vi "GFITS_GetHeaderArray.vi"(0 "file":path, 5 "mext":bool, 7 "number of Extensions":u16, 9 "readmode":string, 11 "error in (no error)":errorcluster, 12 "def_timing":string="after", 13 "headers":bool=TRUE) -> (4 "number of before":i32[](array[numeric]), 6 "After keys":string[][][](array[string]), 8 "number of after keywords":i32[](array[numeric]), 10 "totkeys":i32, 14 "before Keywords":string[][][](array[string]), 15 "error out":errorcluster)   [LabVIEW 2016]
uses:
  DBSHAND/private/vis/DatabaseHand_RefNum.ctl
  GFITS_Gbls.vi
panel:
  in  "Database RefNum in":T1
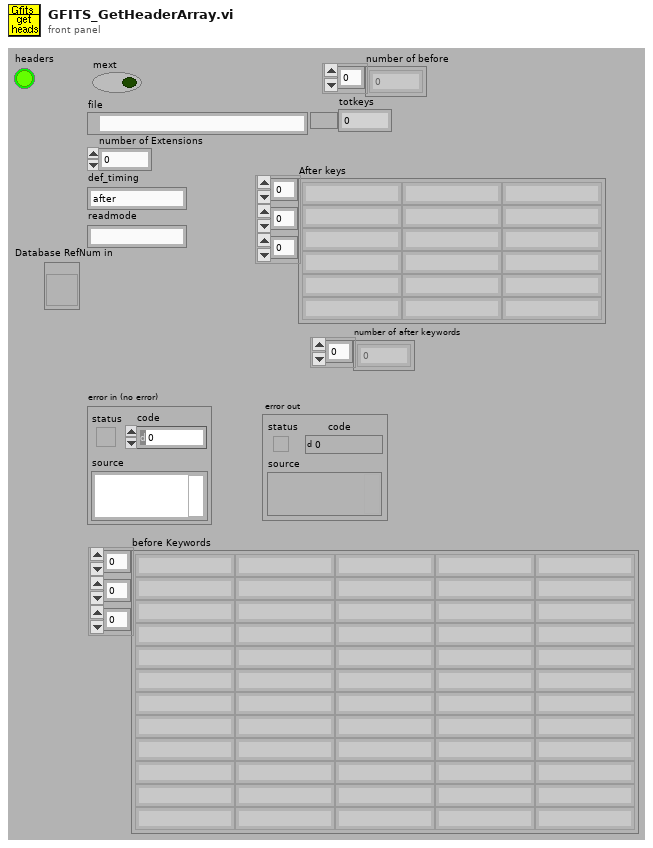
[diagram p1: front panel]
types:
  T1 = typedef "DatabaseHand_RefNum.ctl" = refnum<vi>
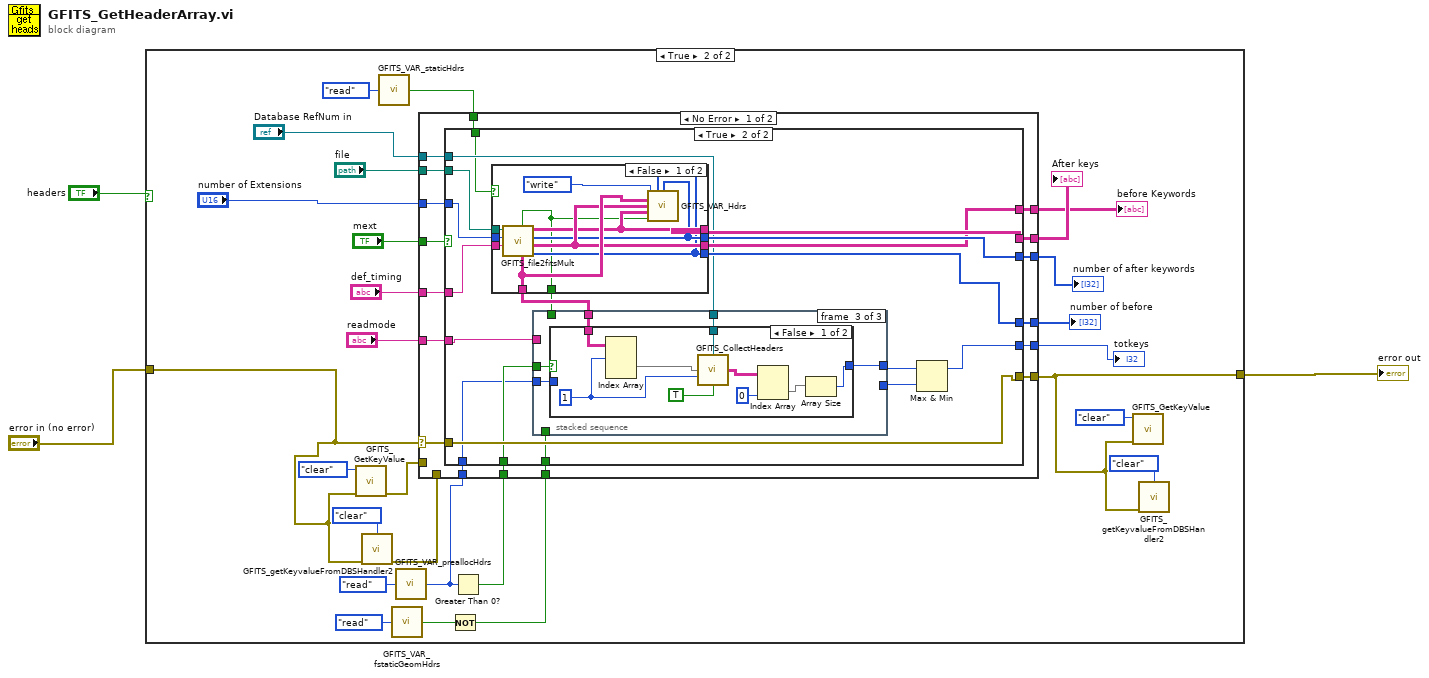
[diagram p0: block diagram]
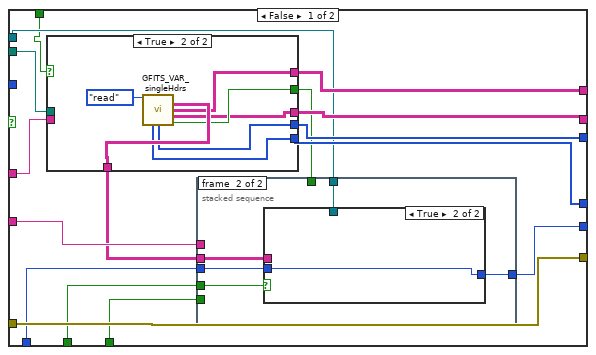
[diagram p3: hidden frame]
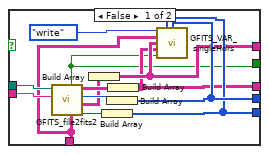
[diagram p4: hidden frame]
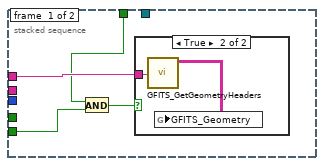
[diagram p5: hidden frame]
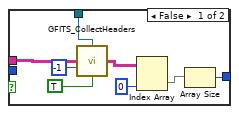
[diagram p7: hidden frame]
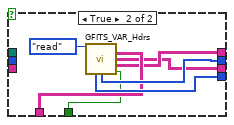
[diagram p8: hidden frame]
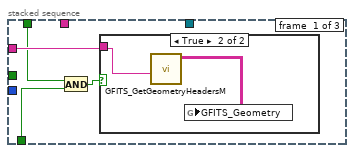
[diagram p9: hidden frame]
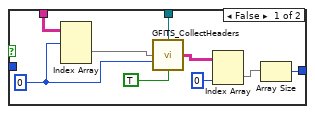
[diagram p12: hidden frame]
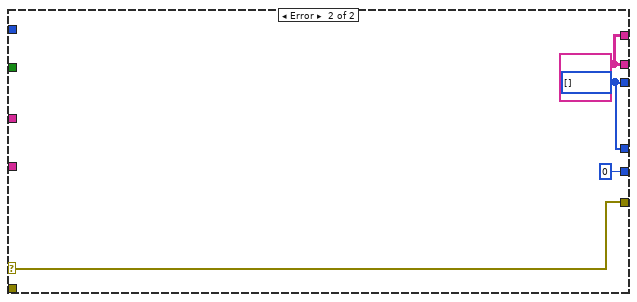
[diagram p14: hidden frame]
diagram:
  n1 = case shown="True" "headers" {
    tunnel: "error in (no error)" -> [w4 w7]
    tunnel: [w4 w19] -> w2
    frame False {
    }
    frame True {
      n2 = call "GFITS_GetKeyValue.vi"("error in (no error)"=w7, "action"=enum16{"get", "clear"}."clear") -> ("error out"=w21:errorcluster)  [unwired: 1 in, 8 out]
      n3 = call "GFITS_getKeyvalueFromDBSHandler2.vi"("action"=enum16{"get", "clear"}."clear", "error in (no error)"=w7) -> ("error out"=w20:errorcluster)  [unwired: 7 in, 6 out]
      n4 = call "GFITS_VAR_staticHdrs.vi"("action"=enum16{"read", "write"}."read") -> ("static out"=w12:bool)  [unwired: 1 in, 13 out]
      n5 = call "GFITS_VAR_fstaticGeomHdrs.vi"("action"=enum16{"read", "write"}."read") -> ("static out"=w9:bool)  [unwired: 1 in, 13 out]
      n6 = call "GFITS_VAR_preallocHdrs.vi"("action"=enum16{"read", "write"}."read") -> ("nkeys out"=w13:i32)  [unwired: 1 in, 13 out]
      n7 = Not(x=w9) -> (.not. x?=w8:bool)
      n8 = Greater Than 0?(x=w13) -> (x > 0?=w14:bool)
      n9 = case shown="No Error" w7 {
        selector: w7 -> [w40 w180]
        tunnel: "mext" -> [w48 _]
        tunnel: "file" -> [w47 _]
        tunnel: "number of Extensions" -> [w46 _]
        tunnel: "def_timing" -> [w45 _]
        tunnel: "readmode" -> [w44 _]
        tunnel: [w43 w177] -> w27
        tunnel: [w42 w179] -> w26
        tunnel: [w41 w180] -> w19
        tunnel: w21 -> [_ _]
        tunnel: w20 -> [_ _]
        tunnel: [w39 w179] -> w18
        tunnel: [w38 0 ("number of total keywords")] -> w6
        tunnel: [w37 w177] -> w17
        tunnel: "Database RefNum in" -> [w36 _]
        tunnel: w12 -> [w35 _]
        tunnel: w14 -> [w34 _]
        tunnel: w13 -> [w33 _]
        tunnel: w8 -> [w32 _]
        frame No Error {
          n10 = case shown="True" w48 {
            tunnel: [w64 w123] -> w43
            tunnel: [w63 w117] -> w42
            tunnel: w47 -> [w62 w122]
            tunnel: w46 -> [_ w119]
            tunnel: w45 -> [w61 w121]
            tunnel: w44 -> [w60 w120]
            tunnel: w40 -> [w59 w118]
            tunnel: [w59 w118] -> w41
            tunnel: [w58 w116] -> w39
            tunnel: [w54 w110] -> w38
            tunnel: [w57 w115] -> w37
            tunnel: w36 -> [w55 w114]
            tunnel: w35 -> [w52 w108]
            tunnel: w34 -> [w51 w107]
            tunnel: w33 -> [w50 w106]
            tunnel: w32 -> [w49 w105]
            frame False {
              n11 = case shown="True" w52 {
                tunnel: [w66 w80] -> w64
                tunnel: [w70 w78] -> w63
                tunnel: w62 -> [w75 _]
                tunnel: w61 -> [w74 _]
                tunnel: [w69 w79] -> w58
                tunnel: [w67 w81] -> w57
                tunnel: [w68 w83] -> w56
                tunnel: [w65 w82] -> w53
                frame False {
                  n12 = call "GFITS_file2fits2.vi"("def_timing"=w74, "file"=w75) -> ("number of before keywords"=w73:i32, "before Keywords"=w72:string[][], "number of after keywords"=w76:i32, "after Keywords"=w77:string[][], "all keys"=w68:string[][], "geominfo?"=w65:bool)  [unwired: 4 out]
                  n13 = Build Array(w72) -> (w67:string[][][])
                  n14 = Build Array(w73) -> (w69:i32[])
                  n15 = Build Array(w76) -> (w70:i32[])
                  n16 = Build Array(w77) -> (w66:string[][][])
                  n17 = call "GFITS_VAR_singleHdrs.vi"("action"=enum16{"read", "write"}."write", "nkeys before in"=w69, "nkeys after in"=w70, "GFITS_allkeys in"=w68, "GFITS_beforein"=w67, "GFITS_after in"=w66, "geom info in"=w65) -> ()  [unwired: 9 out]
                }
                frame True {
                  n18 = call "GFITS_VAR_singleHdrs.vi"("action"=enum16{"read", "write"}."read") -> ("GFITS_allkeys"=w83:string[][], "GFITS_before"=w81:string[][][], "GFITS_after"=w80:string[][][], "nkeys before"=w79:i32[], "nkeys after"=w78:i32[], "geom info"=w82:bool)  [unwired: 6 in, 3 out]
                }
              }
              n19 = stacked-sequence {
                tunnel: w60 -> [w88 _]
                tunnel: w56 -> [_ w95]
                tunnel: w55 -> [_ w94]
                tunnel: [_ w93] -> w54
                tunnel: w53 -> [w85 _]
                tunnel: w51 -> [_ w92]
                tunnel: w50 -> [_ w91]
                tunnel: w49 -> [w86 _]
                frame #0 {
                  n20 = And(x=w85, y=w86) -> (x .and. y?=w87:bool)
                  n21 = case shown="True" w87 {
                    tunnel: w88 -> [_ w90]
                    frame False {
                    }
                    frame True {
                      n22 = call "GFITS_GetGeometryHeaders.vi"("readmode"=w90) -> ("Keywords out"=w89:string[][][])  [unwired: 10 out]
                      n23 = global write "GFITS_Gbls.vi" "GFITS_Geometry"(w89) -> ()
                    }
                  }
                }
                frame #1 {
                  n24 = case shown="True" w92 {
                    tunnel: w95 -> [w103 _]
                    tunnel: w94 -> [w102 _]
                    tunnel: [w96 w104] -> w93
                    tunnel: w91 -> [_ w104]
                    frame False {
                      n25 = call "GFITS_CollectHeaders.vi"("Database RefNum in"=w102, "Keywords"=w103, "extension"=i16 -1, "nd queue"=TRUE) -> ("headers"=w99:string[][])  [unwired: 1 in, 10 out]
                      n26 = Index Array(array=w99, index (col)=0 ("disabled index (col)")) -> (element=w97:string[])  [unwired: 1 in]
                      n27 = Array Size(array=w97) -> (size(s)=w96:i32)
                    }
                    frame True {
                    }
                  }
                }
              }
            }
            frame True {
              n28 = case shown="False" w108 {
                tunnel: [w127 w135] -> w123
                tunnel: w122 -> [w133 _]
                tunnel: w121 -> [w132 _]
                tunnel: w119 -> [w131 _]
                tunnel: [w126 w139] -> w117
                tunnel: [w125 w138] -> w116
                tunnel: [w128 w134] -> w115
                tunnel: [w129 w137] -> w113
                tunnel: [w124 w136] -> w109
                frame False {
                  n29 = call "GFITS_file2fitsMult.vi"("def_timing"=w132, "number of Extensions"=w131, "filename"=w133) -> ("number of before keys"=w125:i32[], "before keys"=w128:string[][][], "number of keywords"=w126:i32[], "Keywords"=w127:string[][][], "all keys"=w129:string[][][], "geominfo?"=w124:bool)  [unwired: 1 in, 2 out]
                  n30 = call "GFITS_VAR_Hdrs.vi"("action"=enum16{"read", "write"}."write", "nkeys before in"=w125, "nkeys after in"=w126, "GFITS_allkeys in"=w129, "GFITS_beforein"=w128, "GFITS_after in"=w127, "geom info in"=w124) -> ()  [unwired: 9 out]
                }
                frame True {
                  n31 = call "GFITS_VAR_Hdrs.vi"("action"=enum16{"read", "write"}."read") -> ("GFITS_allkeys"=w137:string[][][], "GFITS_before"=w134:string[][][], "GFITS_after"=w135:string[][][], "nkeys before"=w138:i32[], "nkeys after"=w139:i32[], "geom info"=w136:bool)  [unwired: 6 in, 3 out]
                }
              }
              n32 = stacked-sequence {
                tunnel: w120 -> [w144 _ _]
                tunnel: w114 -> [_ w151 w166]
                tunnel: w113 -> [_ w150 w165]
                tunnel: [_ w149 _] -> w111
                tunnel: [_ _ w164] -> w112
                tunnel: w109 -> [w143 _ _]
                tunnel: w107 -> [_ w148 w163]
                tunnel: w106 -> [_ w147 w162]
                tunnel: w105 -> [w141 _ _]
                frame #0 {
                  n33 = And(x=w143, y=w141) -> (x .and. y?=w142:bool)
                  n34 = case shown="True" w142 {
                    tunnel: w144 -> [_ w146]
                    frame False {
                    }
                    frame True {
                      n35 = call "GFITS_GetGeometryHeadersM.vi"("readmode"=w146) -> ("Keywords out"=w145:string[][][])  [unwired: 10 out]
                      n36 = global write "GFITS_Gbls.vi" "GFITS_Geometry"(w145) -> ()
                    }
                  }
                }
                frame #1 {
                  n37 = case shown="True" w148 {
                    tunnel: w151 -> [w156 _]
                    tunnel: w150 -> [w155 _]
                    tunnel: [w152 w161] -> w149
                    tunnel: w147 -> [_ w161]
                    frame False {
                      w153 = i16 0 ("extension")
                      n38 = Index Array(array=w155, index (dim 0)=w153) -> (element=w154:string[][])  [unwired: 2 in]
                      n39 = call "GFITS_CollectHeaders.vi"("Database RefNum in"=w156, "Keywords"=w154, "extension"=w153, "nd queue"=TRUE) -> ("headers"=w159:string[][])  [unwired: 1 in, 10 out]
                      n40 = Index Array(array=w159, index (col)=0 ("disabled index (col)")) -> (element=w157:string[])  [unwired: 1 in]
                      n41 = Array Size(array=w157) -> (size(s)=w152:i32)
                    }
                    frame True {
                    }
                  }
                }
                frame #2 {
                  n42 = case shown="False" w163 {
                    tunnel: w166 -> [w171 _]
                    tunnel: w165 -> [w170 _]
                    tunnel: [w167 w176] -> w164
                    tunnel: w162 -> [_ w176]
                    frame False {
                      w168 = i16 1 ("extension")
                      n43 = Index Array(array=w170, index (dim 0)=w168) -> (element=w169:string[][])  [unwired: 2 in]
                      n44 = call "GFITS_CollectHeaders.vi"("Database RefNum in"=w171, "Keywords"=w169, "extension"=w168, "nd queue"=TRUE) -> ("headers"=w174:string[][])  [unwired: 1 in, 10 out]
                      n45 = Index Array(array=w174, index (col)=0 ("disabled index (col)")) -> (element=w172:string[])  [unwired: 1 in]
                      n46 = Array Size(array=w172) -> (size(s)=w167:i32)
                    }
                    frame True {
                    }
                  }
                }
              }
              n47 = Max & Min(x=w112, y=w111) -> (max(x,y)=w110:i32)  [unwired: 1 out]
            }
          }
        }
        frame Error {
          w177 = string[][][] [] ("Keywords")
          w179 = i32[] [] ("number of keywords")
        }
      }
      "number of after keywords" <- w26
      "After keys" <- w27
      "totkeys" <- w6
      "number of before" <- w18
      "before Keywords" <- w17
      n48 = call "GFITS_GetKeyValue.vi"("error in (no error)"=w19, "action"=enum16{"get", "clear"}."clear") -> ()  [unwired: 1 in, 9 out]
      n49 = call "GFITS_getKeyvalueFromDBSHandler2.vi"("action"=enum16{"get", "clear"}."clear", "error in (no error)"=w19) -> ()  [unwired: 7 in, 7 out]
    }
  }
  "error out" <- w2
